vi "TDTSyn-Get Events (Client Side).vi"(0 "IP Address":string, 5 "Port":i32, 7 "last read":bool, 11 "error in (no error)":errorcluster) -> (4 "Codes":i16[](array[numeric]), 8 "Times":sgl[](array[numeric]), 15 "error out":errorcluster)   [LabVIEW 2020]
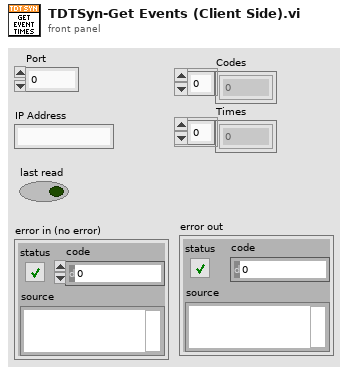
[diagram p1: front panel]
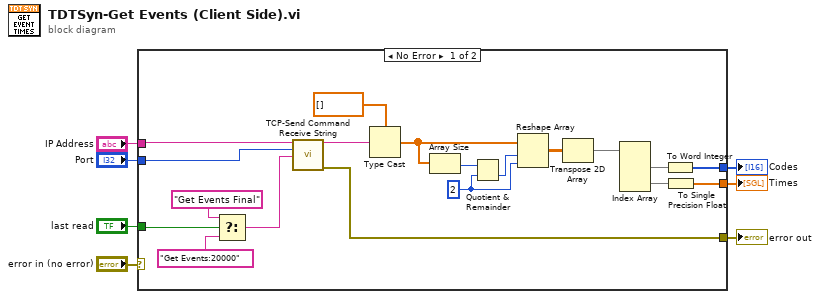
[diagram p0: block diagram]
diagram:
  n1 = case shown="No Error" "error in (no error)" {
    selector: "error in (no error)" -> [_ w27]
    tunnel: "IP Address" -> [w24 _]
    tunnel: "Port" -> [w23 _]
    tunnel: "last read" -> [w26 _]
    tunnel: [w20 w27] -> w3
    tunnel: [w10 _] -> w2
    tunnel: [w9 _] -> w1
    frame No Error {
      w15 = 2 ("dimension size")
      n2 = Select(t="Get Events Final" ("Command"), s=w26, f="Get Events:20000" ("Command")) -> (s? t:f=w8:string)
      n3 = call "TCP-Send Command Receive String.vi"("PXI Address"=w24, "Port"=w23, "Command"=w8) -> ("data"=w22:string, "error out"=w20:errorcluster)  [unwired: 11 in]
      n4 = Type Cast(type=dbl[] [], x=w22) -> (*(type *) &x=w14:dbl[])
      n5 = Array Size(array=w14) -> (size(s)=w17:i32)
      n6 = Quotient & Remainder(x=w17, y=w15) -> (floor(x/y)=w16:i32)  [unwired: 1 out]
      n7 = Reshape Array(w14, w16, w15) -> (w18:dbl[][])
      n8 = Transpose 2D Array(2D array=w18) -> (transposed array=w13:dbl[][])
      n9 = Index Array(array=w13) -> (element #1=w12:dbl[], element #2=w11:dbl[])  [unwired: 4 in]
      n10 = To Word Integer(number=w12) -> (16bit integer=w10:i16[])
      n11 = To Single Precision Float(number=w11) -> (single precision float=w9:sgl[])
    }
    frame Error {
    }
  }
  "error out" <- w3
  "Codes" <- w2
  "Times" <- w1
